vi "Kinect_Example.vi"() -> ()   [LabVIEW 2015]
doc: "Simple demonstration of the Kinesthesia toolkit which allows user to conect the Kinect sensor to LabVIEW"
uses:
  <vilib>/University of Leeds/Kinesthesia Toolkit for Microsoft Kinect/_Polymorphic Configure/Event-Skeleton and Video.vi
  <vilib>/University of Leeds/Kinesthesia Toolkit for Microsoft Kinect/_Polymorphic Read/Read-Skeleton and Video.vi
  <vilib>/University of Leeds/Kinesthesia Toolkit for Microsoft Kinect/_Polymorphic Close/Close-Skeleton and Video.vi
panel:
  out "2D Picture":picture
  out "3D Skeleton":refnum<vi>(3d-picture)
  in  "stop":bool
  # "Kinect - Capture Skeleton Example"
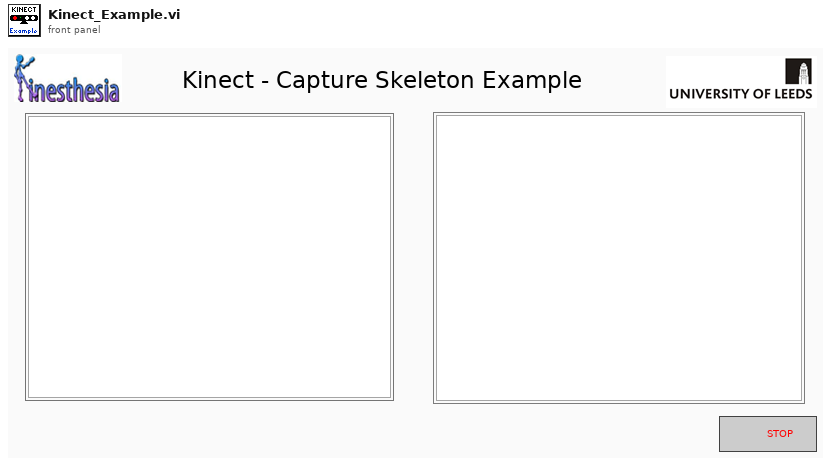
[diagram p1: front panel]
types:
  T1 = cluster{cluster{"reference out":refnum<k24>, "KinectSensors":refnum<k24>}, "get_Item":refnum<k24>}
  T2 = cluster{"reference out":refnum<k24>, "KinectSensors":refnum<k24>, "SkeletonStream":refnum<k24>, "ColorStream":refnum<k24>, refnum<k24>[], "get_Item":refnum<k24>}
  T3 = cluster{"Scene":refnum<vi>, "Joints":refnum<vi>[], "Bones":refnum<vi>[]}
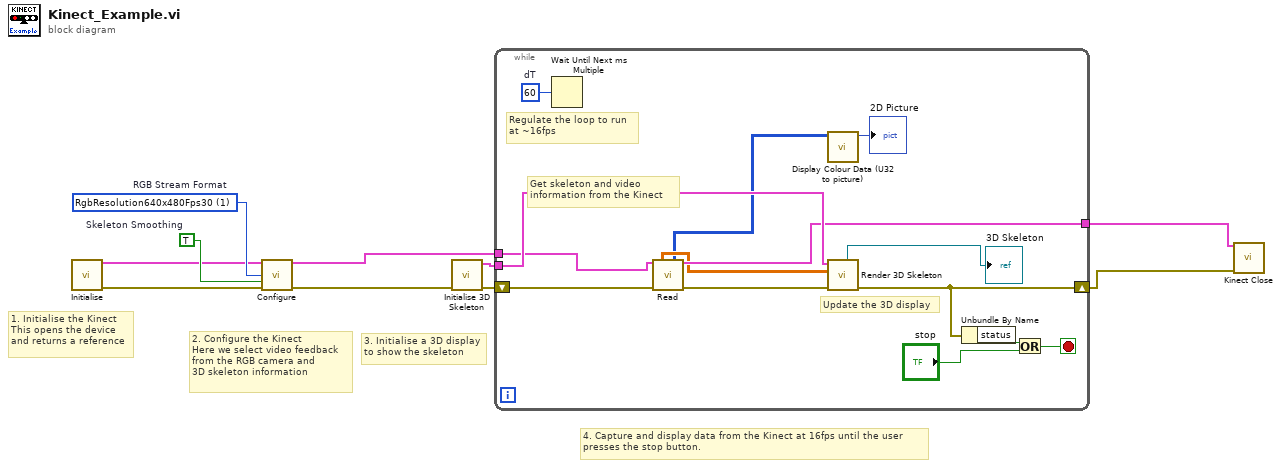
[diagram p0: block diagram]
diagram:
  w6 = 1 items=["Undefined", "RgbResolution640x480Fps30", "RgbResolution1280x960Fps12", "YuvResolution640x480Fps15", "RawYuvResolution640x480Fps15"]  # RGB Stream Format
  w5 = TRUE  # Skeleton Smoothing
  # "4. Capture and display data from the Kinect at 16fps until the user\npresses the stop button."
  # "3. Initialise a 3D display\nto show the skeleton"
  # "2. Configure the Kinect\nHere we select video feedback\nfrom the RGB camera and \n3D skeleton information"
  # "1. Initialise the Kinect\nThis opens the device\nand returns a reference"
  n1 = call <vilib>:"Initialise.vi"() -> ("Kinect References out"=w1:T1, "error out"=w2:errorcluster)  [unwired: 14 in]
  n2 = call-poly <vilib>:"Configure.vi"("Kinect References in"=w1, "RGB Stream Format"=w6, "Skeleton Smoothing"=w5, "error in"=w2) -> ("Kinect References out"=w7:T2, "error out"=w8:errorcluster)  [unwired: 10 in]
  n3 = call <vilib>:"Initialise 3D Skeleton.vi"("error in (no error)"=w8) -> ("error out"=w9:errorcluster, "Scene & Skeleton Refs"=w10:T3)  [unwired: 9 in]
  n4 = while {
    tunnel: [w13] -> w3
    tunnel: w10 -> [w24]
    tunnel: w7 -> [w14]
    shift-right: [w16] -> w4
    shift-left: w9 -> [w20]
    stop <- w17 stop-if-true
    w22 = u32 60  # dT
    # "Update the 3D display"
    # "Get skeleton and video\ninformation from the Kinect"
    # "Regulate the loop to run\nat ~16fps"
    n5 = Wait Until Next ms Multiple(millisecond multiple=w22) -> ()  [unwired: 1 out]
    n6 = call-poly <vilib>:"Read.vi"("Kinect References in"=w14, "error in (no error)"=w20) -> ("Primary Skeleton Array"=w12:dbl[][], "Colour output array (U24, RGB)"=w11:u32[][], "Kinect References out"=w13:T2, "error out"=w19:errorcluster)  [unwired: 9 in, 1 out]
    n7 = call <vilib>:"Display Colour Data (U32 to picture).vi"("Colour output array (U24, RGB)"=w11) -> ("new picture"=→"2D Picture":picture)  [unwired: 10 in]
    n8 = call <vilib>:"Render 3D Skeleton.vi"("error in (no error)"=w19, "Array of Joint Positions"=w12, "Scene & Skeleton Refs In"=w24) -> ("error out"=w16:errorcluster, "Scene Out"=→"3D Skeleton":refnum<vi>)  [unwired: 5 in, 2 out]
    n9 = Unbundle By Name(w16) -> ("status"=w15:bool)
    n10 = Or(x=w15, y="stop") -> (x .or. y?=w17:bool)
  }
  n11 = call-poly <vilib>:"Kinect Close.vi"("Kinect References in"=w3, "error in"=w4) -> ()  [unwired: 13 in, 1 out]
